vi "Get Wavelength.vi"(7 "Ref Wavelength":refnum<vi>, 8 "error in":errorcluster, 9 "Head Channel":i16, 10 "Pulsar Handle":i16, 11 "OphirFastX (in)":refnum<k7>) -> (0 "error out":errorcluster, 3 "OphirFastX (out)":refnum<k7>)   [LabVIEW 2009]
panel:
  # "Guillaume Plateau - yguig2@yahoo.fr"
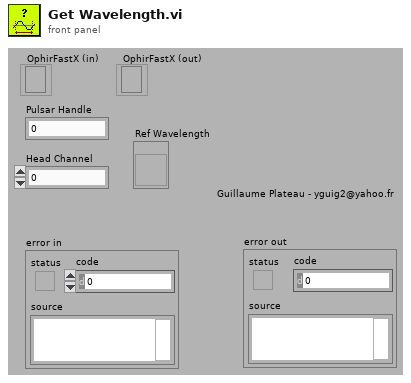
[diagram p1: front panel]
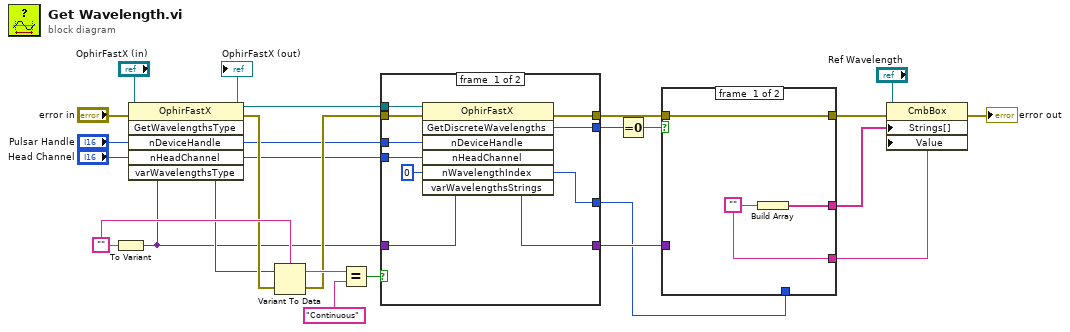
[diagram p0: block diagram]
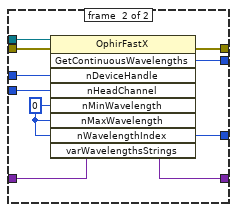
[diagram p2: hidden frame]
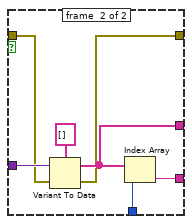
[diagram p3: hidden frame]
diagram:
  w21 = ""
  n1 = To Variant(anything=w21) -> (Variant=w11:variant)
  n2 = invoke class="OphirFastX" method="GetWavelengthsType"(reference="OphirFastX (in)", error in="error in", "nDeviceHandle"="Pulsar Handle", "nHeadChannel"="Head Channel", "varWavelengthsType"=w11) -> (reference out=w16:refnum<k7>, error out=w20:errorcluster, "nDeviceHandle"=w13:i16, "nHeadChannel"=w12:i16, "varWavelengthsType"=w19:variant)  [unwired: 1 in, 1 out]
  "OphirFastX (out)" <- w16
  n3 = Variant To Data(error in=w20, Variant=w19, type=w21) -> (error out=w14:errorcluster, data=w17:string)
  n4 = Equal?(x=w17, y="Continuous") -> (x = y?=w15:bool)
  n5 = case shown="True" w15 {
    tunnel: w16 -> [w35 w45]
    tunnel: w14 -> [w34 w44]
    tunnel: w13 -> [w33 w43]
    tunnel: w12 -> [w32 w42]
    tunnel: w11 -> [w30 w40]
    tunnel: [w28 w39] -> w10
    tunnel: [w29 w38] -> w8
    tunnel: [w27 w37] -> w7
    tunnel: [w26 w36] -> w6
    frame #0 {
      n6 = invoke class="OphirFastX" method="GetDiscreteWavelengths"(reference=w35, error in=w34, "nDeviceHandle"=w33, "nHeadChannel"=w32, "nWavelengthIndex"=i16 0, "varWavelengthsStrings"=w30) -> (error out=w29:errorcluster, "GetDiscreteWavelengths"=w28:i32, "nWavelengthIndex"=w26:i16, "varWavelengthsStrings"=w27:variant)  [unwired: 1 in, 3 out]
    }
    frame #1 {
      w41 = i16 0 ("nMinWavelength")
      n7 = invoke class="OphirFastX" method="GetContinuousWavelengths"(reference=w45, error in=w44, "nDeviceHandle"=w43, "nHeadChannel"=w42, "nMinWavelength"=w41, "nMaxWavelength"=w41, "nWavelengthIndex"=w41, "varWavelengthsStrings"=w40) -> (error out=w38:errorcluster, "GetContinuousWavelengths"=w39:i32, "nWavelengthIndex"=w36:i16, "varWavelengthsStrings"=w37:variant)  [unwired: 1 in, 5 out]
    }
  }
  n8 = Equal To 0?(x=w10) -> (x = 0?=w9:bool)
  n9 = case shown="True" w9 {
    tunnel: w7 -> [_ w55]
    tunnel: w8 -> [w46 w54]
    tunnel: [w48 w52] -> w1
    tunnel: [w47 w51] -> w3
    tunnel: [w46 w50] -> w4
    tunnel: w6 -> [_ w49]
    frame #0 {
      w47 = ""
      n10 = Build Array(w47) -> (w48:string[])
    }
    frame #1 {
      n11 = Variant To Data(error in=w54, Variant=w55, type=string[] []) -> (error out=w50:errorcluster, data=w52:string[])
      n12 = Index Array(array=w52, index=w49) -> (element=w51:string)
    }
  }
  n13 = property class="CmbBox"(reference="Ref Wavelength", error in=w4, "Strings[]"=w1, "Value"=w3) -> (error out=→"error out":errorcluster)  [unwired: 1 out]
